vi "zad3.vi"(8 "error in (no error)":errorcluster, 11 "N":dbl) -> (0 "error out":errorcluster, 3 "Array":dbl[](array[numeric]))   [LabVIEW 2017]
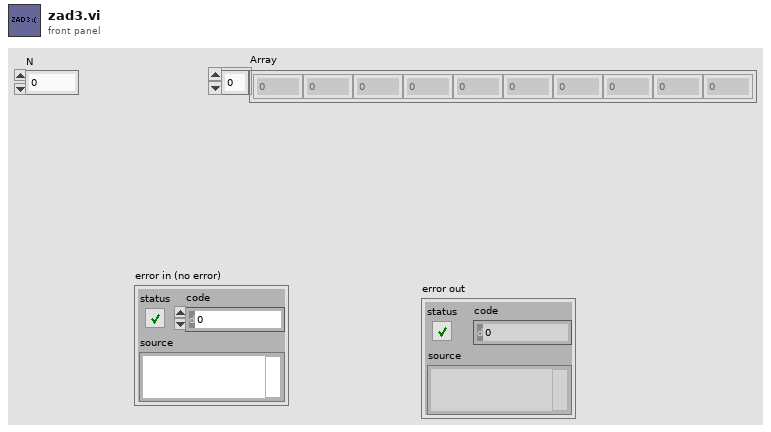
[diagram p1: front panel]
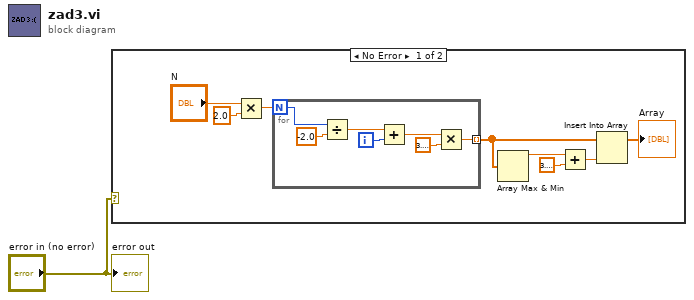
[diagram p0: block diagram]
diagram:
  n1 = case shown="No Error" "error in (no error)" {
    frame No Error {
      n2 = Multiply(x="N", y=2.0 ("Numeric")) -> (x*y=w7:dbl)
      n3 = for {
        N: w7 -> [w11]
        tunnel: [w12] -> w5 mode=indexing
        i -> [w10]
        n4 = Divide(x=w11, y=-2.0 ("Numeric")) -> (x/y=w15:dbl)
        n5 = Add(x=w15, y=w10) -> (x+y=w13:dbl)
        n6 = Multiply(x=w13, y=3.141592653589793) -> (x*y=w12:dbl)
      }
      n7 = Array Max & Min(array=w5) -> (max value=w3:dbl)  [unwired: 3 out]
      n8 = Add(x=w3, y=3.141592653589793) -> (x+y=w2:dbl)
      n9 = Insert Into Array(array=w5, new element=w2) -> (→"Array":dbl[])  [unwired: 1 in]
    }
    frame Error {
    }
  }
  "error out" <- "error in (no error)"
